vi "地址索引.vi"(8 "error in (no error)":errorcluster caption="错误输入（无错误）", 10 "values":u16[](array[numeric]), 11 "测量参数":u16(ring) items=["总磷"=1, "总氮"=2, "氨氮"=3, "COD"=22]) -> (0 "error out":errorcluster caption="错误输出", 3 "MB session out":refnum<class "MB_Master.lvclass">)   [LabVIEW 2016, in "斯坦道总氮.lvlib"]
uses:
  <vilib>/Plasmionique/MB Master/MB_Master/MB_Master.lvclass
  <vilib>/Plasmionique/MB Master/MB Master.lvlib
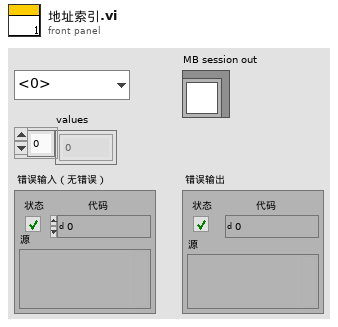
[diagram p1: front panel]
types:
  T1 = typedef "Semaphore RefNum" = refnum<k1>
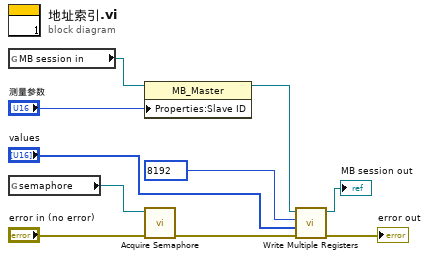
[diagram p0: block diagram]
diagram:
  n1 = global read "VAR总磷总氮全局变量.vi" "MB session in"() -> (w6:refnum<class "MB_Master.lvclass">)
  n2 = global read "VAR总磷总氮全局变量.vi" "semaphore"() -> (w2:T1)
  n3 = property class="MB_Master"(reference=w6, "Properties:Slave ID"="测量参数") -> (reference out=w10:refnum<class "MB_Master.lvclass">)  [unwired: 1 in, 1 out]
  n4 = call <vilib>:"Acquire Semaphore.vi"("error in (no error)"="error in (no error)", "semaphore"=w2) -> ("error out"=w4:errorcluster)  [unwired: 3 in, 2 out]
  n5 = call <vilib>:"Write Multiple Registers.vi"("error in (no error)"=w4, "values"="values", "starting address"=u16 8192, "MB session in"=w10) -> ("error out"=→"error out":errorcluster, "MB session out"=→"MB session out":refnum<class "MB_Master.lvclass">)  [unwired: 6 in]
